vi "send_result.vi"(7 "JSON Tree In (JSON Object)":variant, 8 "error in":errorcluster, 9 "timeout ms":i32, 10 "result":variant, 11 "connection ID":refnum<k5>) -> (0 "error out":errorcluster, 1 "bytes":string, 2 "#bytes written":i32, 3 "connection ID out":refnum<k5>)   [LabVIEW 2010]
uses:
  i3-json-1.0.0-10/JSON Generation/Create Value Files/Create Value - Object.vi
  i3-json-1.0.0-10/JSON Generation/Add Object Parameter Files/Add Object Parameter - Known Type.vi
  i3-json-1.0.0-10/JSON Parsing/Get Object Parameter Files/Get Object Parameter - String.vi
  i3-json-1.0.0-10/JSON Generation/Add Object Parameter Files/Add Object Parameter - String.vi
  i3-json-1.0.0-10/JSON Generation/Add Object Parameter Files/Add Object Parameter - Boolean.vi
  i3-json-1.0.0-10/i3-json.lvlib
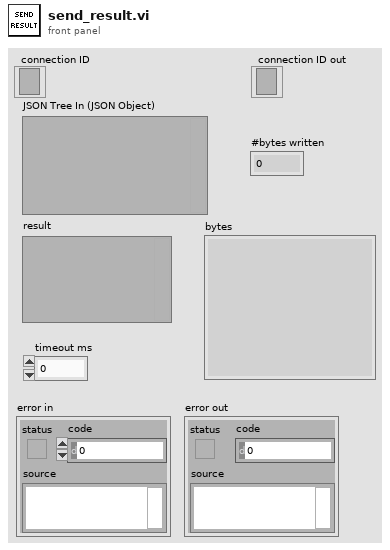
[diagram p1: front panel]
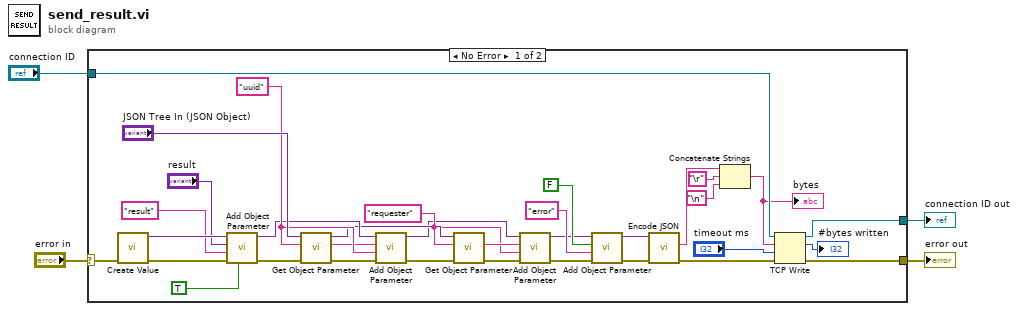
[diagram p0: block diagram]
diagram:
  n1 = case shown="No Error" "error in" {
    selector: "error in" -> [w9 w40]
    tunnel: "connection ID" -> [w37 w39]
    tunnel: [w36 w40] -> w3
    tunnel: [w34 w39] -> w2
    frame No Error {
      w23 = "uuid" ("name")
      w16 = "requester" ("name")
      n2 = call-poly "Create Value.vi"("error in (no error)"=w9) -> ("error out"=w7:errorcluster, "JSON Tree"=w29:variant)  [unwired: 9 in]
      n3 = call-poly "Add Object Parameter.vi"("Add Parameter as JSON Tree?"=TRUE, "error in (no error)"=w7, "Name"="result" ("Default Value if JSON Null"), "Value"="result", "JSON Tree in (JSON Object)"=w29) -> ("error out"=w25:errorcluster, "JSON Tree out (JSON Object)"=w21:variant)  [unwired: 5 in]
      n4 = call-poly "Get Object Parameter.vi"("error in (no error)"=w25, "Parameter Name"=w23, "JSON Tree In (JSON Object)"="JSON Tree In (JSON Object)") -> ("error out"=w24:errorcluster, "String Value"=w22:string, "JSON Tree Out Passthrough"=w17:variant)  [unwired: 5 in, 1 out]
      n5 = call-poly "Add Object Parameter.vi"("error in (no error)"=w24, "Name"=w23, "String"=w22, "JSON Tree in (JSON Object)"=w21) -> ("error out"=w18:errorcluster, "JSON Tree out (JSON Object)"=w15:variant)  [unwired: 6 in]
      n6 = call-poly "Get Object Parameter.vi"("error in (no error)"=w18, "Parameter Name"=w16, "JSON Tree In (JSON Object)"=w17) -> ("error out"=w19:errorcluster, "String Value"=w20:string)  [unwired: 5 in, 2 out]
      n7 = call-poly "Add Object Parameter.vi"("error in (no error)"=w19, "Name"=w16, "String"=w20, "JSON Tree in (JSON Object)"=w15) -> ("error out"=w14:errorcluster, "JSON Tree out (JSON Object)"=w11:variant)  [unwired: 6 in]
      n8 = call-poly "Add Object Parameter.vi"("error in (no error)"=w14, "Name"="error", "Boolean"=FALSE, "JSON Tree in (JSON Object)"=w11) -> ("error out"=w10:errorcluster, "JSON Tree out (JSON Object)"=w6:variant)  [unwired: 6 in]
      n9 = call "Encode JSON.vi"("error in (no error)"=w10, "JSON Tree"=w6) -> ("error out"=w27:errorcluster, "String"=w33:string)  [unwired: 4 in]
      n10 = Concatenate Strings(w33, "\r", "\n") -> (w30:string)
      "bytes" <- w30
      n11 = TCP Write(connection ID=w37, data in=w30, error in (no error)=w27, 9:"timeout ms") -> (connection ID out=w34:refnum<k5>, bytes written=→"#bytes written":i32, error out=w36:errorcluster)
    }
    frame Error {
    }
  }
  "error out" <- w3
  "connection ID out" <- w2
